vi "Find Changed Connections Array Element.vi"(8 "error in (no error)":errorcluster, 10 "OldVal":T2[](array[typedef]), 11 "NewVal":T2[](array[typedef])) -> (0 "error out":errorcluster, 1 "Array Index":i32, 2 "Element Changed":T1)   [LabVIEW 2017, in "Routing and Faulting System Explorer.lvlib"]
uses:
  Routing and Faulting System Explorer.lvlib
  Connection Row.ctl
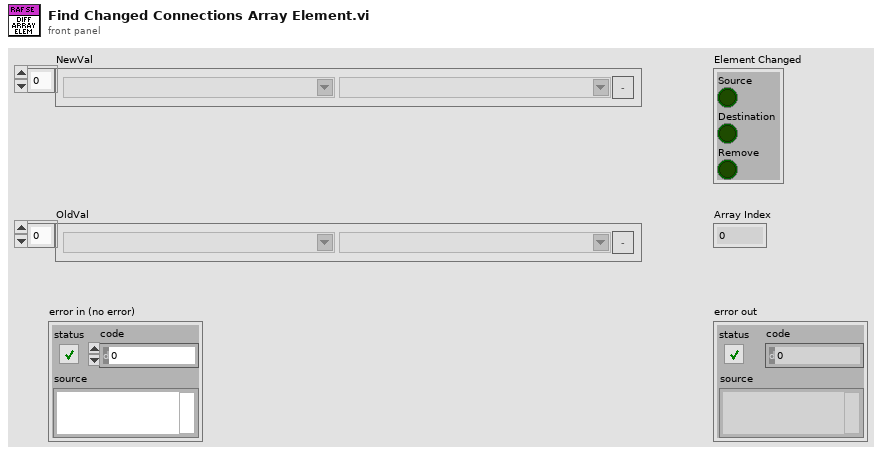
[diagram p1: front panel]
types:
  T1 = cluster{"Source":bool, "Destination":bool, "Remove":bool}
  T2 = typedef "Routing and Faulting System Explorer.lvlib/Connection Row.ctl" = cluster{"Source":string, "Destination":string, "Remove":bool}
  T3 = cluster{"Source":bool, "Destination":bool, "Remove":bool}[]
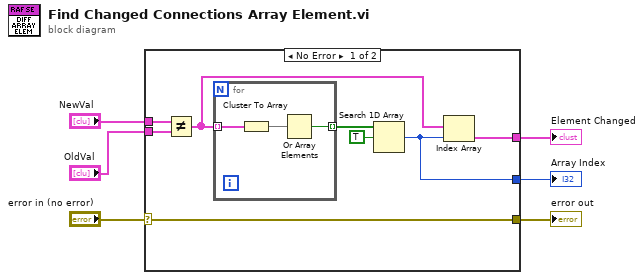
[diagram p0: block diagram]
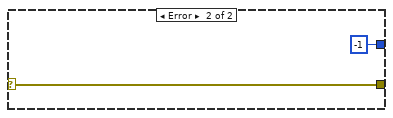
[diagram p2: hidden frame]
diagram:
  n1 = case shown="No Error" "error in (no error)" {
    selector: "error in (no error)" -> [w7 w19]
    tunnel: [w12 -1 ("index of element")] -> w6
    tunnel: "NewVal" -> [w10 _]
    tunnel: "OldVal" -> [w9 _]
    tunnel: [w8 _] -> w3
    tunnel: [w7 w19] -> w1
    frame No Error {
      n2 = Not Equal?(x=w10, y=w9) -> (x != y?=w11:T3)
      n3 = for {
        tunnel: w11 -> [w15] mode=indexing
        tunnel: [w16] -> w14 mode=indexing
        n4 = Cluster To Array(cluster=w15) -> (array=w17:bool[])
        n5 = Or Array Elements(Boolean array=w17) -> (logical OR=w16:bool)
      }
      n6 = Search 1D Array(1D array=w14, element=TRUE) -> (index of element=w12:i32)  [unwired: 1 in]
      n7 = Index Array(array=w11, index=w12) -> (element=w8:T1)
    }
    frame Error {
    }
  }
  "error out" <- w1
  "Array Index" <- w6
  "Element Changed" <- w3
